vi "Measurement Logic.vi"() -> ()   [LabVIEW 2024, in "NIFgenSignalVoltageGeneration.lvlib"]
uses:
  NIFgenSignalVoltageGeneration.lvlib
  Measurement Results.ctl
  <instrlib>/niFgen/niFgen.llb/niFgen Output Mode.ctl
  <vilib>/MeasurementLink/MeasurementLink Session Management V1/Session Reservation/Session Reservation.lvclass
  <vilib>/MeasurementLink/MeasurementLink niFGEN/MeasurementLink niFGEN.lvlib
  <vilib>/MeasurementLink/MeasurementLink Measurement Server/Measure Call Context/Measure Call Context.lvclass
  <vilib>/MeasurementLink/MeasurementLink niFGEN/Initialize Sessions - 1Sess.vi
  <instrlib>/niFgen/niFgen.llb/niFgen Waveform Type.ctl
  Measurement Configuration.ctl
panel:
  out "Generated Waveform":waveform(dbl)(graph)
  out "measure call context out":refnum<class "Measure Call Context.lvclass">
  in  "measure call context in":refnum<class "Measure Call Context.lvclass">
  out "measurement results":T1
  in  "measurement configuration":T2={"Pin Name"="Pin1", "Generation Time (s)"=0.0, "Voltage Offset (V)"=0.0, "Sample Rate (Hz)"=1000000.0, "Frequency (Hz)"=200000.0, "Amplitude (Vpk-pk)"=1.0, "Waveform"=0} {"Waveform" items=["Sine"=0, "Square"=3]}
  out "error out":errorcluster
  in  "error in":errorcluster
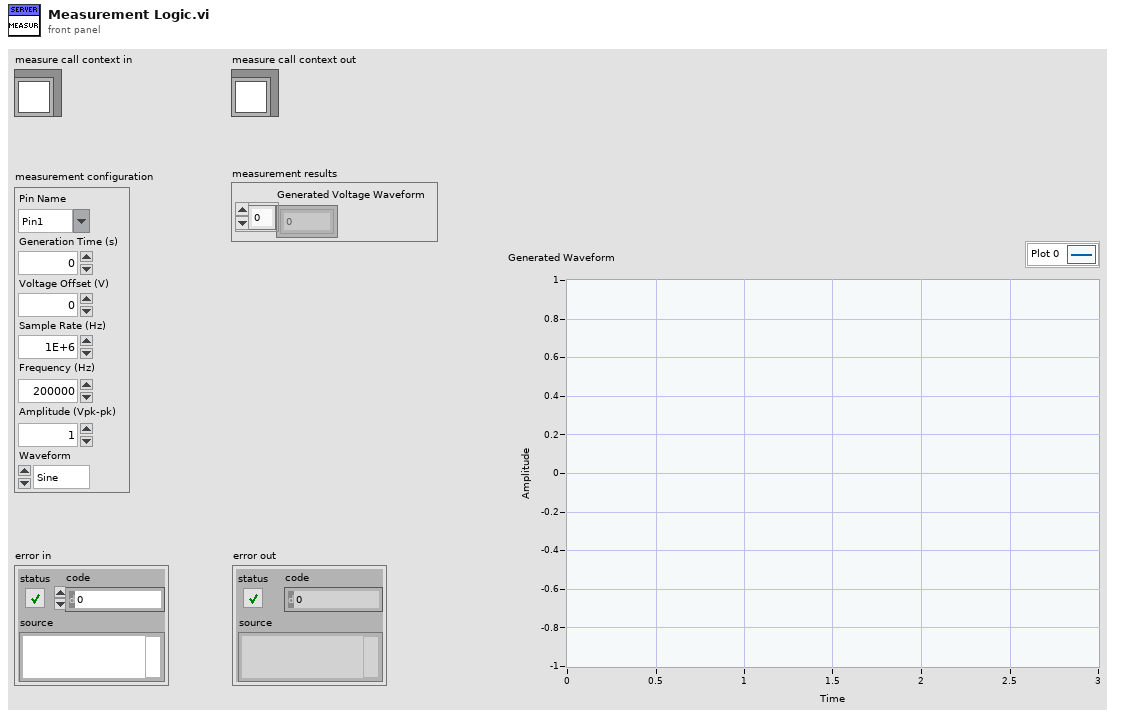
[diagram p1: front panel]
types:
  T1 = typedef "NIFgenSignalVoltageGeneration.lvlib/Measurement Results.ctl" = cluster{"Generated Voltage Waveform":dbl[]}
  T2 = typedef "NIFgenSignalVoltageGeneration.lvlib/Measurement Configuration.ctl" = cluster{"Pin Name":string, "Generation Time (s)":dbl, "Voltage Offset (V)":dbl, "Sample Rate (Hz)":dbl, "Frequency (Hz)":dbl, "Amplitude (Vpk-pk)":dbl, "Waveform":i32}
  T3 = typedef "niFgen Output Mode.ctl" = u32
  T4 = cluster{"Waveform":i32, "Amplitude (Vpk-pk)":dbl, dbl}
  T5 = typedef "niFgen Waveform Type.ctl" = i32
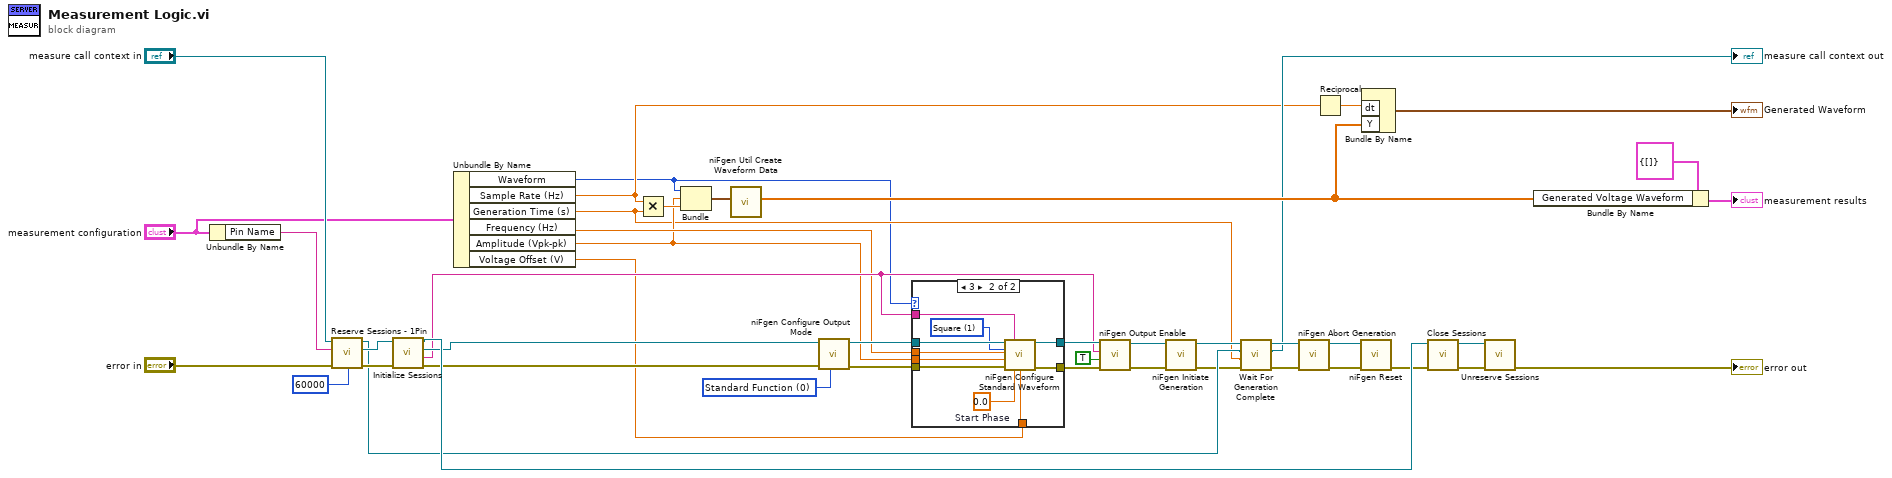
[diagram p0: block diagram]
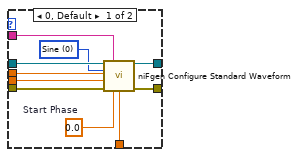
[diagram p2: hidden frame]
diagram:
  w39 = T3 0 items=["Standard Function", "Frequency List", "Arbitrary Waveform", "Arbitrary Sequence", "Script"] ("Output Mode (default: 0=Standard Function)")
  n1 = Unbundle By Name("measurement configuration") -> ("Pin Name"=w19:string)
  n2 = call <vilib>:"Reserve Sessions - 1Pin.vi"("timeout (ms)"=60000, "error in"="error in", "pin or relay name"=w19, "measurement context in"="measure call context in") -> ("error out"=w42:errorcluster, "session reservation out"=w41:refnum<class "Session Reservation.lvclass">, "measurement context out"=w9:refnum<class "Measure Call Context.lvclass">)  [unwired: 5 in]
  n3 = call-poly <vilib>:"Initialize Sessions.vi"("error in"=w42, "session reservation in"=w41) -> ("error out"=w35:errorcluster, "channel list"=w23:string, "session"=w34:refnum<k15>, "session reservation out"=w36:refnum<class "Session Reservation.lvclass">)  [unwired: 6 in]
  n4 = Unbundle By Name("measurement configuration") -> ("Waveform"=w1:i32, "Sample Rate (Hz)"=w2:dbl, "Generation Time (s)"=w6:dbl, "Frequency (Hz)"=w17:dbl, "Amplitude (Vpk-pk)"=w16:dbl, "Voltage Offset (V)"=w15:dbl)
  n5 = Multiply(x=w2, y=w6) -> (x*y=w22:dbl)
  n6 = Bundle("Waveform"=w1, "Amplitude (Vpk-pk)"=w16, w22) -> (w21:T4)  [unwired: 1 in]
  n7 = call <instrlib>:"niFgen Util Create Waveform Data.vi"("Waveform"=w21) -> ("Waveform Data"=w14:dbl[])  [unwired: 10 in]
  n8 = call <instrlib>:"niFgen Configure Output Mode.vi"("error in (no error)"=w35, "Output Mode (default: 0=Standard Function)"=w39, "Instrument Handle"=w34) -> ("error out"=w26:errorcluster, "Instrument Handle Out"=w27:refnum<k15>)  [unwired: 6 in]
  n9 = case shown="3" w1 {
    tunnel: w27 -> [w54 w63]
    tunnel: w26 -> [w45 w62]
    tunnel: [w51 w61] -> w25
    tunnel: [w50 w60] -> w24
    tunnel: w23 -> [w46 w59]
    tunnel: w17 -> [w53 w58]
    tunnel: w16 -> [w52 w57]
    tunnel: w15 -> [w49 w56]
    frame 0, Default {
      w47 = T5 0 items=["Sine", "Square", "Triangle", "Ramp Up", "Ramp Down", "DC", "Noise", "User"] ("Waveform")
      w48 = 0.0  # Start Phase
      n10 = call <instrlib>:"niFgen Configure Standard Waveform.vi"("Instrument Handle"=w54, "Channel Name"=w46, "Waveform"=w47, "Frequency"=w53, "Amplitude"=w52, "error in (no error)"=w45, "Start Phase"=w48, "DC Offset"=w49) -> ("Instrument Handle Out"=w51:refnum<k15>, "error out"=w50:errorcluster)  [unwired: 6 in]
    }
    frame 3 {
      w55 = T5 1 items=["Sine", "Square", "Triangle", "Ramp Up", "Ramp Down", "DC", "Noise", "User"] ("Waveform")
      w64 = 0.0  # Start Phase
      n11 = call <instrlib>:"niFgen Configure Standard Waveform.vi"("Instrument Handle"=w63, "Channel Name"=w59, "Waveform"=w55, "Frequency"=w58, "Amplitude"=w57, "error in (no error)"=w62, "Start Phase"=w64, "DC Offset"=w56) -> ("Instrument Handle Out"=w61:refnum<k15>, "error out"=w60:errorcluster)  [unwired: 6 in]
    }
  }
  n12 = call <instrlib>:"niFgen Output Enable.vi"("error in (no error)"=w24, "Output Enable (default: True)"=TRUE, "Channel Name"=w23, "Instrument Handle"=w25) -> ("error out"=w30:errorcluster, "Instrument Handle Out"=w29:refnum<k15>)  [unwired: 6 in]
  n13 = call <instrlib>:"niFgen Initiate Generation.vi"("error in (no error)"=w30, "Instrument Handle"=w29) -> ("error out"=w8:errorcluster, "Instrument Handle Out"=w10:refnum<k15>)  [unwired: 8 in]
  n14 = call "Wait For Generation Complete.vi"("error in"=w8, "duration"=w6, "measurement context in"=w9, "instrument handle in"=w10) -> ("error out"=w7:errorcluster, "measurement context out"=→"measure call context out":refnum<class "Measure Call Context.lvclass">, "instrument handle out"=w5:refnum<k15>)  [unwired: 4 in, 1 out]
  n15 = call <instrlib>:"niFgen Abort Generation.vi"("error in (no error)"=w7, "Instrument Handle"=w5) -> ("error out"=w32:errorcluster, "Instrument Handle Out"=w33:refnum<k15>)  [unwired: 8 in]
  n16 = Reciprocal(x=w2) -> (1/x=w3:dbl)
  n17 = call <instrlib>:"niFgen Reset.vi"("error in (no error)"=w32, "Instrument Handle"=w33) -> ("error out"=w31:errorcluster)  [unwired: 8 in, 1 out]
  n18 = Bundle By Name("dt"=w3, "Y"=w14) -> (→"Generated Waveform":waveform(dbl))  [unwired: 1 in]
  n19 = call <vilib>:"Close Sessions.vi"("error in"=w31, "session reservation in"=w36) -> ("error out"=w37:errorcluster, "session reservation out"=w38:refnum<class "Session Reservation.lvclass">)  [unwired: 8 in]
  n20 = call <vilib>:"Unreserve Sessions.vi"("error in"=w37, "session reservation in"=w38) -> ("error out"=→"error out":errorcluster)  [unwired: 9 in]
  n21 = Bundle By Name(cluster=T1 {"Generated Voltage Waveform"=[]} ("Measurement Results"), "Generated Voltage Waveform"=w14) -> (→"measurement results":T1)
